vi "Seq_Stop.vi"(8 "error in (no error)":errorcluster) -> (0 "error out":errorcluster)   [LabVIEW 2016, in "SeqProcessor.lvlib"]
uses:
  SeqProcessor.lvlib
  controls/Flag.ctl
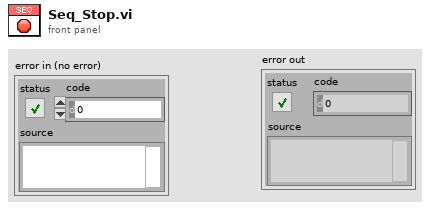
[diagram p1: front panel]
types:
  T1 = typedef "SeqProcessor.lvlib/Flag.ctl" = cluster{"SingleStep":bool, "Pause":bool, "Stop":bool, "StepbyStep":bool}
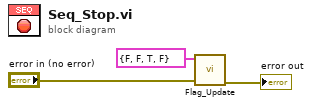
[diagram p0: block diagram]
diagram:
  n1 = call "Flag_Update.vi"("error in (no error)"="error in (no error)", "Flag"=T1 {"SingleStep"=FALSE, "Pause"=FALSE, "Stop"=TRUE, "StepbyStep"=FALSE}) -> ("error out"=→"error out":errorcluster)  [unwired: 9 in]
